vi "FTW-Container-New-FromVariant.vi"(5 "Variant":variant, 11 "error in":errorcluster) -> (4 "FTW-Container":refnum<class "FTW-Container.lvclass">, 15 "error out":errorcluster)   [LabVIEW 2015, in "FTW-Container.lvclass"]
uses:
  FTW-Container.lvclass
  <vilib>/Utility/Data Type/NI_Data Type.lvlib
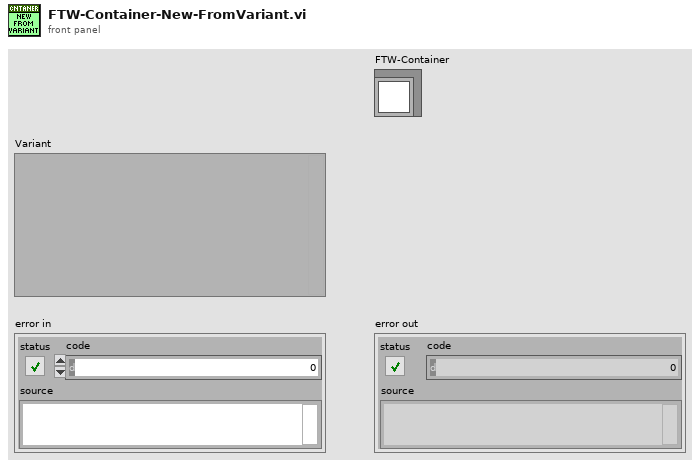
[diagram p1: front panel]
types:
  T1 = typedef "NI_Data Type.lvlib/Data Type.ctl" = enum8{"Invalid Type", "Void", "I8", "I16", "I32", "I64", "U8", "U16", "U32", "U64", "Single Float", "Double Float", "Extended Float", "Single Complex", "Double Complex", "Extended Complex", "Enum U8", "Enum U16", "Enum U32", "Enum U64", "Single Float With Unit", "Double Float With Unit", "Extended Float With Unit", "Single Complex with Unit", "Double Complex with Unit", "Extended Complex with Unit", "Boolean", "String", "Path", "Picture", "Tag", "Array", "Cluster", "Variant", "LV Variant", "Waveform", "Timestamp", "Digital Waveform", "Digital Data", "ExpressData", "Refnum", "External Data", "VI", "Poly VI", "LabVIEW Class Instance", "Fixed Point"}
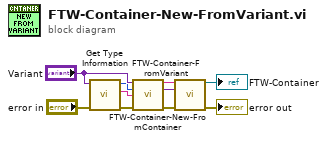
[diagram p0: block diagram]
diagram:
  n1 = call <vilib>:"Get Type Information.vi"("error in (no error)"="error in", "Variant"="Variant") -> ("error out"=w8:errorcluster, "Name"=w6:string, "Type"=w7:T1)  [unwired: 5 in, 2 out]
  n2 = call "FTW-Container-FromVariant.vi"("Variant"="Variant", "Type"=w7, "Name"=w6, "error in"=w8) -> ("Name"=w3:string, "Container"=w2:variant, "error out"=w5:errorcluster)  [unwired: 9 in]
  n3 = call "FTW-Container-New-FromContainer.vi"("Name"=w3, "Container"=w2, "error in"=w5) -> ("FTW-Container"=→"FTW-Container":refnum<class "FTW-Container.lvclass">, "error out"=→"error out":errorcluster)  [unwired: 11 in]
